vi "3 motor init.vi"(6 "Variable PID(Kp)":T2={"Enable variable PID(Kp)"=TRUE, "Variable PID(Kp)range"=0.3, "Variable MODE"=enum."Sin&Cos"}, 7 "Array 2":T1[](array[typedef]), 8 "Error In":errorcluster, 9 "dt(s)":dbl, 10 "PID":cluster{"Kp":dbl, "Ki":dbl, "Kd":dbl}[](array[cluster]), 11 "Array":refnum<class "Motor single.lvclass">[](array[class])) -> (0 "error out":errorcluster, 3 "Object array":refnum<class "Motor single.lvclass">[](array[class]))   [LabVIEW 2019]
uses:
  motor single class/Variable PID(Kp).ctl
  motor single class/Variable PID(Kp) mode enum.ctl
  motor single class/Motor single.lvclass
  motor enum(FPGA).ctl
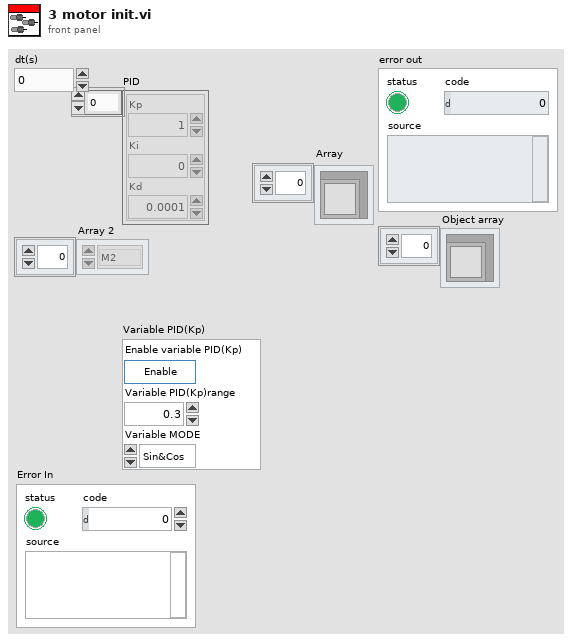
[diagram p1: front panel]
types:
  T1 = typedef "Motor single.lvclass/motor enum(FPGA).ctl" = enum16{"M1", "M2", "M3", "M4"}
  T2 = typedef "Motor single.lvclass/Variable PID(Kp).ctl" = cluster{"Enable variable PID(Kp)":bool, "Variable PID(Kp)range":dbl, "Variable MODE":T3}
  T3 = typedef "Motor single.lvclass/Variable PID(Kp) mode enum.ctl" = enum16{"Log", "Sin&Cos", "Linear", "reverse Log", "const"}
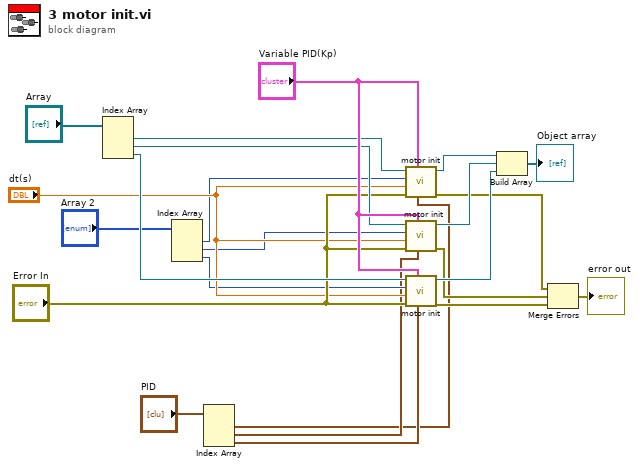
[diagram p0: block diagram]
diagram:
  n1 = Index Array(array="Array") -> (element #1=w21:refnum<class "Motor single.lvclass">, element #2=w20:refnum<class "Motor single.lvclass">, element #3=w19:refnum<class "Motor single.lvclass">)  [unwired: 3 in]
  n2 = Index Array(array="Array 2") -> (element #1=w15:T1, element #2=w14:T1, element #3=w13:T1)  [unwired: 3 in]
  n3 = Index Array(array="PID") -> (element #1=w1:cluster{"Kp":dbl, "Ki":dbl, "Kd":dbl}, element #2=w2:cluster{"Kp":dbl, "Ki":dbl, "Kd":dbl}, element #3=w3:cluster{"Kp":dbl, "Ki":dbl, "Kd":dbl})  [unwired: 3 in]
  n4 = call "motor init.vi"("PID"=w1, "Variable PID(Kp)"="Variable PID(Kp)", "Error In"="Error In", "dt(s)"="dt(s)", "Enum"=w15, "Motor single.lvclass"=w21) -> ("Error Out"=w8:errorcluster, "output object"=w12:refnum<class "Motor single.lvclass">)  [unwired: 4 in]
  n5 = call "motor init.vi"("PID"=w2, "Variable PID(Kp)"="Variable PID(Kp)", "Error In"="Error In", "dt(s)"="dt(s)", "Enum"=w14, "Motor single.lvclass"=w20) -> ("Error Out"=w7:errorcluster, "output object"=w10:refnum<class "Motor single.lvclass">)  [unwired: 4 in]
  n6 = call "motor init.vi"("PID"=w3, "Variable PID(Kp)"="Variable PID(Kp)", "Error In"="Error In", "dt(s)"="dt(s)", "Enum"=w13, "Motor single.lvclass"=w19) -> ("Error Out"=w9:errorcluster, "output object"=w11:refnum<class "Motor single.lvclass">)  [unwired: 4 in]
  n7 = Build Array(w12, w10, w11) -> (→"Object array":refnum<class "Motor single.lvclass">[])
  n8 = Merge Errors(w8, w7, w9) -> (→"error out":errorcluster)
